vi "Init.vi"(8 "error in (no error)":errorcluster, 11 "Mouse in":refnum<class "Mouse.lvclass">) -> (0 "error out":errorcluster, 3 "Mouse out":refnum<class "Mouse.lvclass">)   [LabVIEW 2020, in "Maze.lvlib" / "Mouse.lvclass"]
doc: "Init is called when the mouse is first loaded so it can initialize any references, memory, queues, etc. that it may use in its runs. If this VI is overridden then also be sure to override <i>Cleanup.vi</i> to release these resources.\n\nOne of the objectives of this challenge is to have your mouse navigate a maze it has already run faster on successive runs. This means that this VI is only called once during the lifetime of your mouse to allow it to retain knowledge of previous runs and there are other VIs that can be overridden such as <i>Start.vi</i>, <i>New Maze.vi</i>, and others to know when to reuse or reset maze memory."
uses:
  Mouse.lvclass
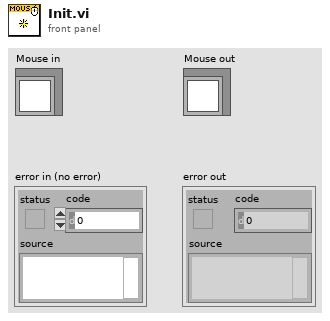
[diagram p1: front panel]
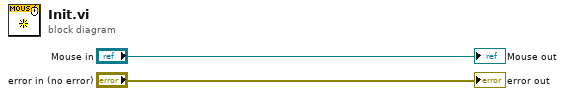
[diagram p0: block diagram]
diagram:
  "error out" <- "error in (no error)"
  "Mouse out" <- "Mouse in"
